vi "ValidateNumInColumn.vi"(8 "Number":i32, 9 "Column":i32, 10 "Row":i32, 11 "Board":i32[][](array[numeric])) -> (0 "Number":i32, 1 "Column":i32, 2 "Row":i32, 3 "Board":i32[][](array[numeric]), 4 "Valid in Column":bool)   [LabVIEW 2023]
doc: "Checks if Number is valid in the current Column\n\nInputs\n- Board: Current Board Configuration\n- Row: Row of current Cell\n- Column: Column of current Cell\n- Number: Number to try out in current Cell\n\nOutputs\n- Board: Current Board Configuration\n- Row: Row of current Cell\n- Column: Column of current Cell\n- Number: Number to try out in current Cell\n- Valid in Column: TRUE if Number is valid in current Column"
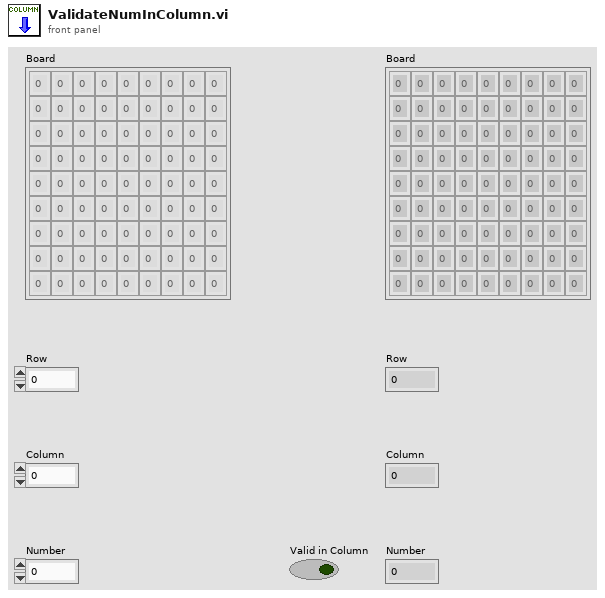
[diagram p1: front panel]
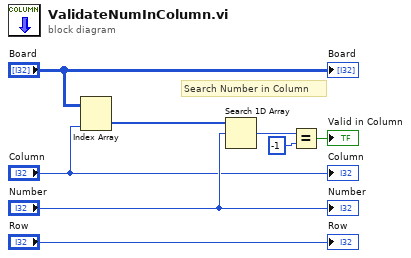
[diagram p0: block diagram]
diagram:
  # "Search Number in Column"
  n1 = Index Array "Index Array"(array="Board", index (col)="Column") -> (element=w4:i32[])  [unwired: 1 in]
  n2 = Search 1D Array(1D array=w4, element="Number") -> (index of element=w3:i32)  [unwired: 1 in]
  n3 = Equal?(x=w3, y=-1) -> (x = y?=→"Valid in Column":bool)
  "Column" <- "Column"
  "Number" <- "Number"
  "Board" <- "Board"
  "Row" <- "Row"
